vi "TDMS Display File.vi"() -> ()   [LabVIEW 2014]
doc: "Reads Channel groups from a storage."
panel:
  in  "Tab Control":enum32{"Graphs", "Text"}(tab)
  out "ADC Graph & Sensitivity":cluster{dbl, dbl, dbl, dbl, dbl}[](graph)=[{0.6939202535855351, 0.6597435304346917, 0.7798494996227666, 0.7113758520027016, 0.041666666666666664}, {0.7732833719705785, 0.6831987858579877, 0.7047989808668466, 0.7000130127327059, 0.041666666666666664}, {0.7041007332325139, 0.6748832071166728, 0.7563758628274665, 0.7023418195101918, 0.041666666666666664}, {0.7287710343361812, 0.6927783915812504, 0.7367118468836872, 0.7748980582895691, 0.041666666666666664}, {0.6905208333838971, 0.747533064441799, 0.7260319680668351, 0.7577968684325942, 0.041666666666666664}, {0.7790184565798852, 0.7089789165824457, 0.7869391330757264, 0.7335479682280418, 0.041666666666666664}, {0.7547574725819008, 0.6794186579039788, 0.7263648203122135, 0.7405852344135999, 0.041666666666666664}, {0.7856012252236705, 0.7164541312349011, 0.7321340500218805, 0.7793940620799212, 0.041666666666666664}, {0.7863694695366785, 0.7192010621853371, 0.7529441881051713, 0.7942795552898763, 0.041666666666666664}, {0.7143802793590173, 0.7267824228941477, 0.7533863587388494, 0.7549754653750381, 0.041666666666666664}, {0.6889570460159845, 0.6978171767970807, 0.752604474645387, 0.7974266882348474, 0.041666666666666664}, {0.7348739186447792, 0.7511512488908724, 0.7862275846371153, 0.7697490282132154, 0.041666666666666664}, {0.7366489816305779, 0.7076468412533097, 0.7941746731939553, 0.7431999420022006, 0.041666666666666664}, {0.7437110525923172, 0.7293183326362236, 0.7328337328163285, 0.7755590941734851, 0.041666666666666664}, {0.754297094768359, 0.7342720364474336, 0.7253119766780587, 0.707530199890292, 0.041666666666666664}, {0.7718793380822023, 0.7305908805566939, 0.777290626488686, 0.7061421406556109, 0.041666666666666664}, {0.7115328838296461, 0.7639583343927541, 0.7103041909758872, 0.7799545729746497, 0.041666666666666664}, {0.7580782799362614, 0.7922444595666327, 0.793582490808957, 0.7164928001393474, 0.041666666666666664}, {0.7209935129318416, 0.7069085518092215, 0.7276454877529765, 0.7347196698830953, 0.041666666666666664}, {0.7072631490766665, 0.7059021200829305, 0.7059235489574393, 0.7928329938510451, 0.041666666666666664}, {0.7558665739764943, 0.783417340400808, 0.7186483662817867, 0.7048531032784096, 0.041666666666666664}, {0.7259888720514239, 0.7827058907882586, 0.7856346509265696, 0.7319576523845315, 0.041666666666666664}, {0.74059829235442, 0.7286867909911054, 0.740318109215077, 0.7529248645791811, 0.041666666666666664}, {0.7356353131734163, 0.7288697068745372, 0.7176850318597146, 0.7717892323258992, 0.041666666666666664}, {0.7173257455525135, 0.7096572295115393, 0.7672636644207551, 0.7931343209935473, 0.041666666666666664}, {0.7728690641585468, 0.7481594582172137, 0.7986948039298276, 0.7227590658562968, 0.041666666666666664}, {0.7240581644010037, 0.7434758157386584, 0.7939639460929329, 0.7796933777948981, 0.041666666666666664}, {0.0, 0.0, 0.0, 0.0, 0.041666666666666664}, {0.0, 0.0, 0.0, 0.0, 0.041666666666666664}, {0.0, 0.0, 0.0, 0.0, 0.041666666666666664}, {0.0, 0.0, 0.0, 0.0, 0.041666666666666664}, {0.0, 0.0, 0.0, 0.0, 0.041666666666666664}, {0.0, 0.0, 0.0, 0.0, 0.041666666666666664}, {0.7755518153902545, 0.7104068769947832, 0.7404803041697349, 0.7571889248547118, 0.041666666666666664}, {0.7149365159428147, 0.7562761667080153, 0.7655658082814235, 0.7546614486574645, 0.041666666666666664}, {0.7212787265758981, 0.7847814585899867, 0.7008701060788964, 0.744848024239413, 0.041666666666666664}, {0.7539590861913611, 0.7362412923320947, 0.7225911968588279, 0.7072678582111586, 0.041666666666666664}, {0.7457332369970215, 0.7772592809738016, 0.7258779848130176, 0.7997742018754828, 0.041666666666666664}, {0.7462202544308557, 0.7595734610688903, 0.7956340843626722, 0.7482255973738333, 0.041666666666666664}, {0.7892949237206847, 0.7338521115039054, 0.7796435247051742, 0.7289646531269393, 0.041666666666666664}, {0.7894512728814828, 0.7582215635979696, 0.7031641919165742, 0.713359715695722, 0.041666666666666664}, {0.7801688183124195, 0.7810196748023058, 0.78113300185513, 0.7321256124215014, 0.041666666666666664}, {0.7724444570393036, 0.7626952195833875, 0.7612535051718013, 0.7636797337587992, 0.041666666666666664}, {0.726193836599923, 0.7025715443395366, 0.7600099653021122, 0.7575978173214227, 0.041666666666666664}, {0.6928599602194575, 0.7798772159854377, 0.7597272438553717, 0.7812075005180638, 0.041666666666666664}, {0.781487809210651, 0.7612062064634987, 0.7218990796443885, 0.7797000424620804, 0.041666666666666664}, {0.7166320541009918, 0.7834263100440512, 0.7678515500809588, 0.7922811439738483, 0.041666666666666664}, {0.7182030947763013, 0.7910931020099308, 0.7851472394092485, 0.7439923396870723, 0.041666666666666664}, {0.6907666179203221, 0.7377810110090649, 0.7810427433401166, 0.7818706862200796, 0.041666666666666664}, {0.7312453712449207, 0.7490604024135352, 0.7532586729256394, 0.7147550021471913, 0.041666666666666664}, {0.7456867608830217, 0.7451360478820621, 0.7931037481358184, 0.767108452826512, 0.041666666666666664}, {0.6951815348463707, 0.7936814204460578, 0.7633267272309218, 0.7942657913383232, 0.041666666666666664}, {0.7553828225357224, 0.7568992495449439, 0.7345922136156305, 0.771588151980189, 0.041666666666666664}, {0.7429695767133445, 0.765897743360358, 0.7634684516022431, 0.7894448586489562, 0.041666666666666664}, {0.7399032091425222, 0.7288032440908395, 0.7303765797296764, 0.7566677502770919, 0.041666666666666664}, {0.7211293560307285, 0.7179158627748919, 0.7554406467422284, 0.7120925129215225, 0.041666666666666664}, {0.7523970348492739, 0.765370991389381, 0.7434740118117725, 0.766108449040928, 0.041666666666666664}, {0.7121501268469138, 0.7925882050278492, 0.751466109048222, 0.7523113271043922, 0.041666666666666664}, {0.7856519081186785, 0.754151490769755, 0.7261868017394744, 0.7186521662932761, 0.041666666666666664}, {0.7761293635703304, 0.7289798730469097, 0.7218306996500045, 0.7038676590417627, 0.041666666666666664}, {0.7179191679481689, 0.7182690162819555, 0.7444122025372735, 0.7067525552015262, 0.041666666666666664}, {0.7391717580052206, 0.7194903373318009, 0.7069946452929429, 0.7628273895478763, 0.041666666666666664}, {0.7528873020695526, 0.7283262360845427, 0.7325000693073801, 0.7327186254922717, 0.041666666666666664}, {0.7627377902903003, 0.7121581200366729, 0.7774356361278989, 0.7864987984211413, 0.041666666666666664}, {0.7614706971450383, 0.7693062686373836, 0.7596520780174131, 0.791453120693149, 0.041666666666666664}, {0.7758676354288726, 0.7329821109544447, 0.7391832844496626, 0.7040621948075004, 0.041666666666666664}, {0.7485651313430548, 0.7218336773536471, 0.7795020189288245, 0.7853101355604608, 0.041666666666666664}, {0.7977503651267112, 0.7593770002282237, 0.7246274031916076, 0.781837212070119, 0.041666666666666664}, {0.7273354149998054, 0.7406129618939882, 0.7473330540821154, 0.7433034517255335, 0.041666666666666664}, {0.7648587772973705, 0.7253507610953411, 0.7915188498462815, 0.7809612467240841, 0.041666666666666664}, {0.7909263018147277, 0.7309183057278329, 0.7000539453979222, 0.701566380552961, 0.041666666666666664}, {0.7719463781719988, 0.7756144498861192, 0.7748605139353143, 0.711833830053124, 0.041666666666666664}, {0.7522821554311848, 0.7941048840894853, 0.7812308538741344, 0.7367902396056907, 0.041666666666666664}, {0.7866854434339422, 0.7904040217561459, 0.786572030675636, 0.7515730253597176, 0.041666666666666664}, {0.7431088687650106, 0.7826296546335783, 0.742585319011906, 0.767182141229277, 0.041666666666666664}, {0.7628229055220703, 0.7520591249139157, 0.7931985520375183, 0.7451458835282231, 0.041666666666666664}, {0.716552177079085, 0.7927089139381129, 0.7577622400472642, 0.7977649378310769, 0.041666666666666664}, {0.708528438337556, 0.707471228807087, 0.7671195999021296, 0.7596502790257245, 0.041666666666666664}, {0.7255377083440769, 0.7283264739729112, 0.7012629971681663, 0.7881931793708195, 0.041666666666666664}, {0.7166590421880428, 0.7183948555292896, 0.7931008558115896, 0.7010772209591309, 0.041666666666666664}, {0.7600625968935042, 0.7244956222335572, 0.752396089672624, 0.7516733687841425, 0.041666666666666664}, {0.71084210554201, 0.735660980564117, 0.7222812162595661, 0.7370424814051276, 0.041666666666666664}, {0.7281773525093489, 0.7025501267298878, 0.7435778600354459, 0.7594209718616234, 0.041666666666666664}, {0.7507708779236648, 0.7466706425110812, 0.7467961834606034, 0.7532602084876552, 0.041666666666666664}, {0.7331378215250902, 0.7690824168048302, 0.7419505671874272, 0.7847182031732947, 0.08333333333333333}, {0.7663900674619695, 0.732831972277527, 0.7091270673435227, 0.704576265161799, 0.125}, {0.7625782253183676, 0.7744159315624022, 0.7836810871865778, 0.77025187606171, 0.03571428571428571}, {0.7662700014377278, 0.7364215860482902, 0.7977560421751317, 0.7046744970371753, 0.019230769230769232}, {0.7023419054532284, 0.7445916524990491, 0.7783197623813431, 0.7718046969464623, 0.017857142857142856}, {0.7940522278437301, 0.7355956777127955, 0.7056827914859263, 0.7699640310025585, 0.03125}, {0.770151412505229, 0.7787470380637564, 0.7701937621436273, 0.7120881251288848, 0.027777777777777776}, {0.7590860680135483, 0.7193515506620416, 0.7482624622113545, 0.7734007737662043, 0.027777777777777776}, {0.7902528716694006, 0.7920635472066051, 0.7061816422974638, 0.7136584188346482, 0.027777777777777776}, {0.7202475273918132, 0.7120728463926694, 0.7099410165077542, 0.7532619723321432, 0.027777777777777776}, {0.7280834311921148, 0.7222543761195239, 0.7752711117539064, 0.7844367655326663, 0.019230769230769232}, {0.7216642070556465, 0.7808386057862613, 0.7269832478590368, 0.7098337925845678, 0.019230769230769232}, {0.7258473468243719, 0.7867000147035547, 0.7901203071285353, 0.7749291489590999, 0.019230769230769232}, {0.7114154074948261, 0.7237034251052005, 0.7768628688354834, 0.7038342654847397, 0.019230769230769232}, {0.776992432147979, 0.7236427920421763, 0.7156948815630676, 0.7884477458876853, 0.013888888888888888}, {0.7827571632521982, 0.7584136008022355, 0.7273492175968963, 0.7662182461929385, 0.013888888888888888}, {0.7183822940750804, 0.746836694478358, 0.7624403222602808, 0.7375898553279964, 0.013888888888888888}, {0.7466792322952455, 0.7752572572433142, 0.7394298853231326, 0.7539515082977921, 0.013888888888888888}, {0.7413928347892835, 0.739015145244675, 0.719535040118229, 0.7995292148267662, 0.013888888888888888}, {0.744576008173865, 0.7435091818234738, 0.7619895596040774, 0.704510502436212, 0.013888888888888888}, {0.7338843271690502, 0.7301459829714548, 0.7516659017287741, 0.7116540086058052, 0.013888888888888888}, {0.7157306194086261, 0.739270530701973, 0.7384527479670627, 0.7635141296986823, 0.013888888888888888}, {0.7927694855533823, 0.7293486704071075, 0.767631027356994, 0.7624067749388849, 0.013888888888888888}, {0.760568663221189, 0.7870702738129487, 0.7180398074034551, 0.7373794865012128, 0.013888888888888888}, {0.0, 0.0, 0.0, 0.0, 0.013888888888888888}]
  out "Motors & Loopback & Clouds":cluster{dbl, dbl, dbl, dbl, dbl, dbl}[](graph)=[{1.0, 0.0, 1.0, 0.0, 1.0, 1.0}, {0.0, 1.0, 0.0, 0.0, 1.0, 1.0}, {1.0, 0.0, 0.0, 0.0, 1.0, 1.0}, {0.0, 0.0, 1.0, 0.0, 1.0, 1.0}, {0.0, 0.0, 0.0, 0.0, 1.0, 1.0}, {0.0, 0.0, 0.0, 0.0, 1.0, 1.0}, {0.0, 0.0, 1.0, 0.0, 1.0, 1.0}, {0.0, 1.0, 1.0, 0.0, 1.0, 1.0}, {0.0, 0.0, 1.0, 0.0, 1.0, 1.0}, {0.0, 0.0, 0.0, 0.0, 1.0, 1.0}, {1.0, 0.0, 1.0, 0.0, 1.0, 1.0}, {1.0, 0.0, 0.0, 0.0, 1.0, 1.0}, {1.0, 0.0, 0.0, 0.0, 1.0, 1.0}, {0.0, 0.0, 1.0, 0.0, 1.0, 1.0}, {0.0, 0.0, 0.0, 0.0, 1.0, 1.0}, {0.0, 0.0, 0.0, 0.0, 1.0, 1.0}, {0.0, 0.0, 0.0, 0.0, 1.0, 1.0}, {0.0, 0.0, 0.0, 1.0, 1.0, 1.0}, {0.0, 0.0, 0.0, 0.0, 1.0, 1.0}, {0.0, 0.0, 0.0, 0.0, 0.0, 1.0}, {0.0, 0.0, 0.0, 0.0, 0.0, 1.0}, {0.0, 0.0, 0.0, 0.0, 0.0, 1.0}, {0.0, 0.0, 0.0, 0.0, 0.0, 1.0}, {0.0, 0.0, 0.0, 0.0, 0.0, 1.0}, {0.0, 0.0, 0.0, 0.0, 0.0, 1.0}, {0.0, 0.0, 0.0, 0.0, 0.0, 1.0}, {0.0, 0.0, 0.0, 0.0, 0.0, 1.0}, {0.0, 0.0, 0.0, 0.0, 0.0, 1.0}, {0.0, 0.0, 0.0, 0.0, 0.0, 1.0}, {0.0, 0.0, 0.0, 0.0, 0.0, 1.0}, {0.0, 0.0, 0.0, 0.0, 0.0, 1.0}, {0.0, 0.0, 0.0, 0.0, 0.0, 1.0}, {0.0, 0.0, 0.0, 0.0, 0.0, 1.0}, {0.0, 0.0, 0.0, 0.0, 0.0, 1.0}, {0.0, 0.0, 0.0, 0.0, 0.0, 1.0}, {0.0, 0.0, 0.0, 0.0, 0.0, 1.0}, {0.0, 0.0, 0.0, 0.0, 0.0, 1.0}, {0.0, 0.0, 0.0, 0.0, 0.0, 1.0}, {0.0, 0.0, 0.0, 0.0, 0.0, 1.0}, {0.0, 0.0, 0.0, 0.0, 0.0, 1.0}, {0.0, 1.0, 0.0, 1.0, 1.0, 1.0}, {0.0, 0.0, 0.0, 1.0, 1.0, 1.0}, {0.0, 0.0, 0.0, 0.0, 1.0, 1.0}, {0.0, 0.0, 1.0, 0.0, 1.0, 1.0}, {1.0, 0.0, 0.0, 0.0, 1.0, 1.0}, {0.0, 1.0, 0.0, 0.0, 1.0, 1.0}, {1.0, 0.0, 0.0, 0.0, 1.0, 1.0}, {1.0, 0.0, 0.0, 1.0, 1.0, 1.0}, {1.0, 0.0, 1.0, 0.0, 1.0, 1.0}, {0.0, 0.0, 0.0, 0.0, 1.0, 1.0}, {1.0, 0.0, 0.0, 0.0, 1.0, 1.0}, {1.0, 0.0, 0.0, 0.0, 1.0, 1.0}, {0.0, 0.0, 0.0, 0.0, 1.0, 1.0}, {0.0, 0.0, 0.0, 0.0, 1.0, 1.0}, {0.0, 0.0, 0.0, 0.0, 1.0, 1.0}, {0.0, 0.0, 0.0, 0.0, 0.0, 1.0}, {0.0, 0.0, 0.0, 0.0, 0.0, 1.0}, {0.0, 0.0, 0.0, 0.0, 0.0, 1.0}, {0.0, 0.0, 0.0, 0.0, 0.0, 1.0}, {0.0, 0.0, 0.0, 0.0, 0.0, 1.0}, {0.0, 0.0, 0.0, 0.0, 0.0, 1.0}, {0.0, 0.0, 0.0, 0.0, 0.0, 1.0}, {0.0, 0.0, 0.0, 0.0, 0.0, 1.0}, {0.0, 0.0, 0.0, 0.0, 0.0, 1.0}, {0.0, 0.0, 0.0, 0.0, 0.0, 1.0}, {0.0, 0.0, 0.0, 0.0, 0.0, 1.0}, {0.0, 0.0, 0.0, 0.0, 0.0, 1.0}, {0.0, 0.0, 0.0, 0.0, 0.0, 1.0}, {0.0, 0.0, 0.0, 0.0, 0.0, 1.0}, {0.0, 0.0, 0.0, 0.0, 0.0, 1.0}, {0.0, 0.0, 0.0, 0.0, 0.0, 1.0}, {0.0, 0.0, 0.0, 0.0, 0.0, 1.0}, {0.0, 0.0, 0.0, 0.0, 0.0, 1.0}, {0.0, 0.0, 0.0, 0.0, 0.0, 1.0}, {0.0, 0.0, 0.0, 0.0, 0.0, 1.0}, {0.0, 0.0, 0.0, 0.0, 0.0, 1.0}, {0.0, 0.0, 0.0, 0.0, 0.0, 1.0}, {0.0, 0.0, 0.0, 0.0, 0.0, 1.0}, {0.0, 0.0, 0.0, 0.0, 0.0, 1.0}, {0.0, 0.0, 0.0, 0.0, 0.0, 1.0}, {0.0, 0.0, 0.0, 0.0, 0.0, 1.0}, {0.0, 0.0, 0.0, 0.0, 0.0, 1.0}, {0.0, 0.0, 0.0, 0.0, 0.0, 1.0}, {0.0, 0.0, 0.0, 0.0, 0.0, 1.0}, {0.0, 0.0, 0.0, 0.0, 0.0, 1.0}, {0.0, 0.0, 0.0, 0.0, 0.0, 1.0}, {0.0, 0.0, 0.0, 0.0, 0.0, 1.0}, {0.0, 0.0, 0.0, 0.0, 0.0, 1.0}, {0.0, 0.0, 0.0, 0.0, 0.0, 1.0}, {0.0, 0.0, 0.0, 0.0, 0.0, 1.0}, {0.0, 0.0, 0.0, 0.0, 0.0, 1.0}, {0.0, 0.0, 0.0, 0.0, 0.0, 1.0}, {0.0, 0.0, 0.0, 0.0, 0.0, 1.0}, {0.0, 0.0, 0.0, 0.0, 0.0, 1.0}, {0.0, 0.0, 0.0, 0.0, 0.0, 1.0}, {0.0, 0.0, 0.0, 0.0, 0.0, 1.0}, {0.0, 0.0, 0.0, 0.0, 0.0, 1.0}, {0.0, 0.0, 0.0, 0.0, 0.0, 1.0}, {0.0, 0.0, 0.0, 0.0, 0.0, 1.0}, {0.0, 0.0, 0.0, 0.0, 0.0, 1.0}, {0.0, 0.0, 0.0, 0.0, 0.0, 1.0}, {0.0, 0.0, 0.0, 0.0, 0.0, 1.0}, {0.0, 0.0, 0.0, 0.0, 0.0, 1.0}, {0.0, 0.0, 0.0, 0.0, 0.0, 1.0}, {0.0, 0.0, 0.0, 0.0, 0.0, 1.0}, {0.0, 0.0, 0.0, 0.0, 0.0, 1.0}, {0.0, 0.0, 0.0, 0.0, 0.0, 1.0}, {0.0, 0.0, 0.0, 0.0, 0.0, 1.0}, {0.0, 0.0, 0.0, 0.0, 0.0, 1.0}]
  out "TIME        ADC0    ADC1    ADC2   ADC3   SENSITIVITY":string[](array[string])
  out "channel name(s)":string[](array[string])
  out "?":variant[](array[variant])
  out "?":string[](array[string])
  # "Original FP"
  # "File properties"
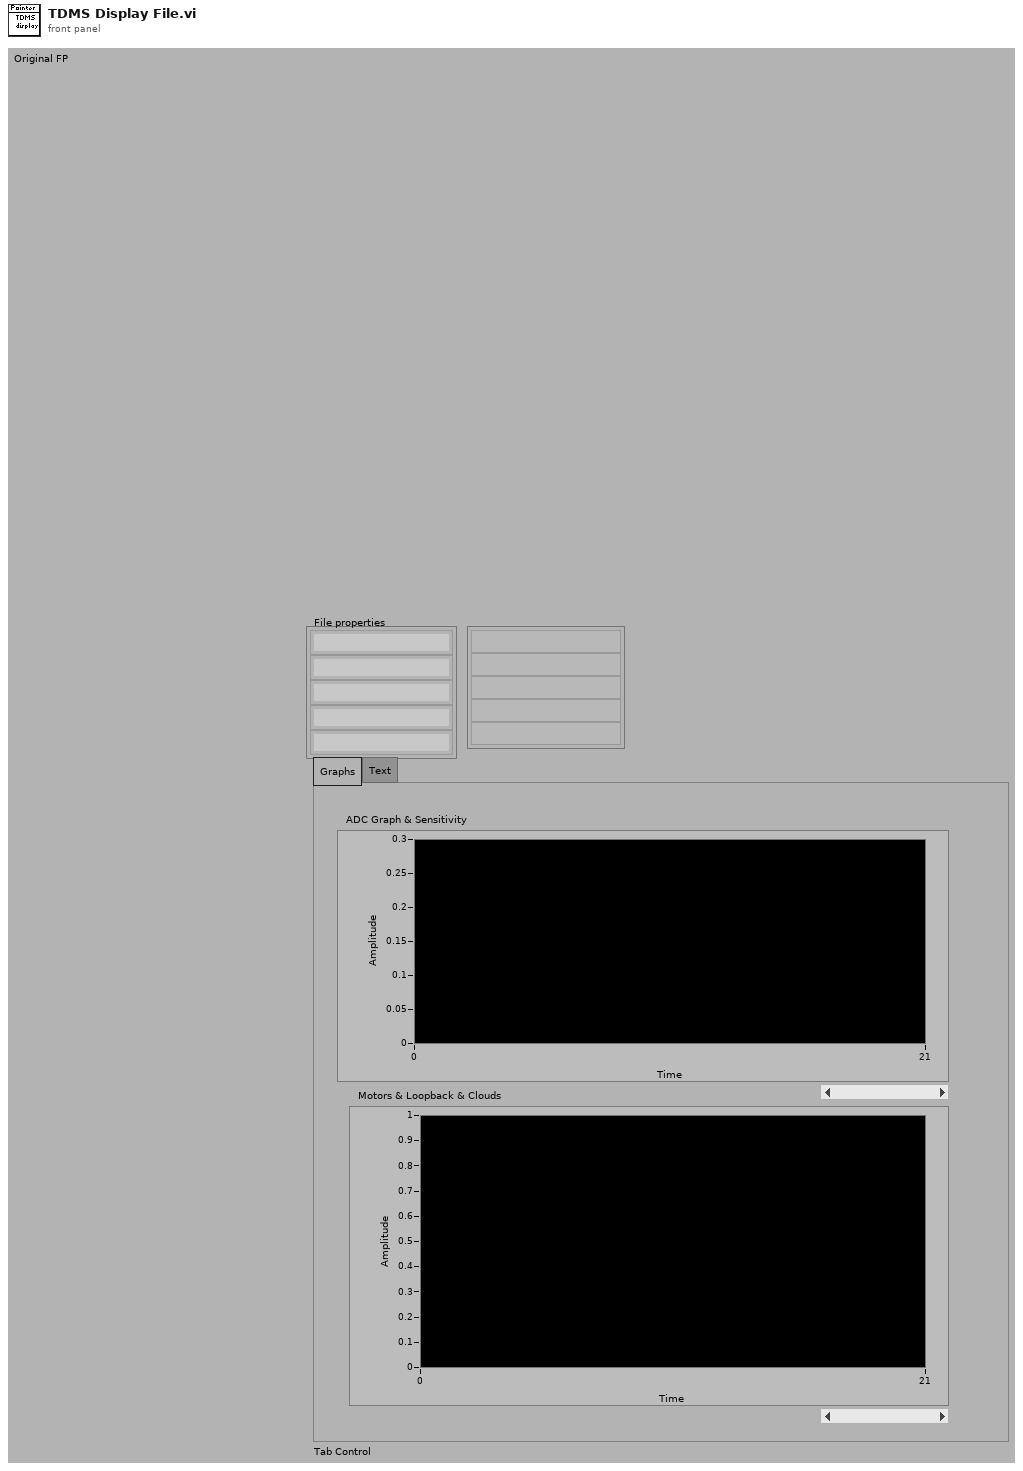
[diagram p1: front panel]
types:
  T1 = enum16{"open", "open or create", "create or replace", "create", "open (read-only)"}
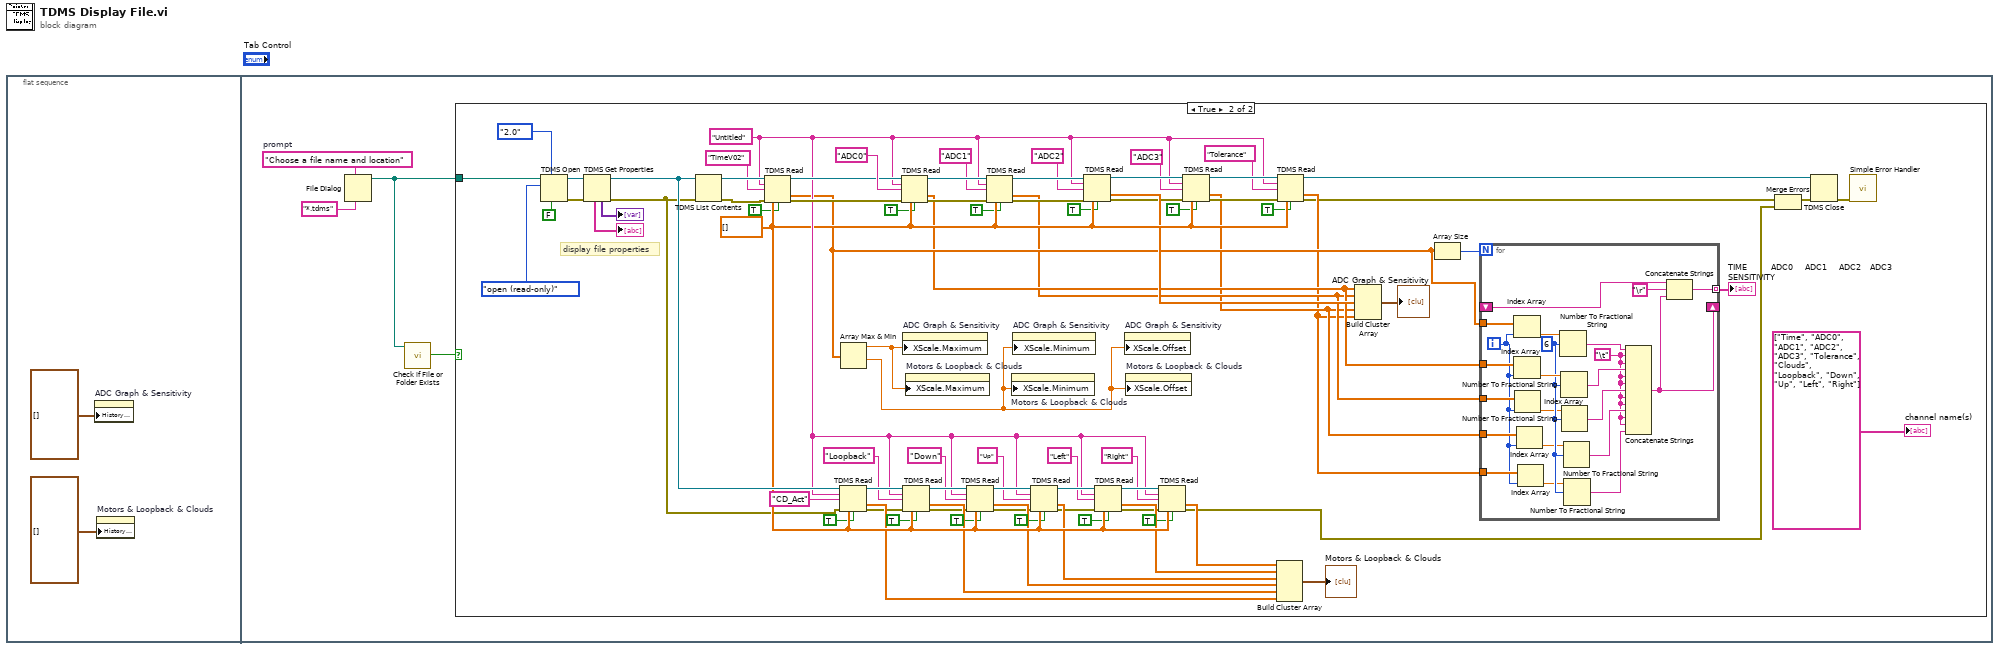
[diagram p0: block diagram]
diagram:
  n1 = flat-sequence {
    frame #0 {
      n2 = property on="ADC Graph & Sensitivity" class="WFChart (strict)"("History Data"=cluster{dbl, dbl, dbl, dbl, dbl}[] []) -> ()  [unwired: 2 in, 2 out]
      n3 = property on="Motors & Loopback & Clouds" class="WFChart (strict)"("History Data"=cluster{dbl, dbl, dbl, dbl, dbl, dbl}[] []) -> ()  [unwired: 2 in, 2 out]
    }
    frame #1 {
      w6 = "Choose a file name and location"  # prompt
      n4 = File Dialog(6:"*.tdms" ("pattern (all files)"), 7:w6) -> (3:w4:path)  [unwired: 1 in, 7 out]
      n5 = call <vilib>:"Check if File or Folder Exists.vi"("path"=w4) -> ("file or folder exists?"=w3:bool)  [unwired: 8 in, 2 out]
      n6 = case shown="True" w3 {
        tunnel: w4 -> [_ w19]
        frame False {
        }
        frame True {
          w48 = dbl[] []
          w54 = "Untitled" ("group name in")
          # "display file properties"
          n7 = TDMS Open(6:FALSE ("disable buffering (T)"), 7:enum16{"1.0", "2.0"}."2.0" ("file format version (2.0)"), 10:T1."open (read-only)" ("operation"), 11:w19) -> (0:w30:errorcluster, 3:w84:refnum<k34>)  [unwired: 3 in]
          n8 = TDMS Get Properties(8:w30, 11:w84) -> (0:w28:errorcluster, 3:w61:refnum<k34>, 4:→"?":variant[], 6:→"?":string[])  [unwired: 6 out]
          n9 = TDMS List Contents(4:w28, 7:w61) -> (0:w73:errorcluster, 3:w81:refnum<k34>)  [unwired: 3 out]
          n10 = TDMS Read(0:w81, 5:w54, 7:"TimeV02" ("channel name(s) in"), 11:w73, 12:w48, 13:TRUE ("return channels in file order? (F)")) -> (4:w67:refnum<k34>, 10:w35:dbl[], 15:w72:errorcluster)  [unwired: 2 in, 3 out]
          n11 = TDMS Read(0:w61, 5:w54, 7:"CD_Act" ("channel name(s) in"), 11:w28, 12:w48, 13:TRUE ("return channels in file order? (F)")) -> (4:w59:refnum<k34>, 10:w42:dbl[], 15:w27:errorcluster)  [unwired: 2 in, 3 out]
          n12 = Array Max & Min(array=w35) -> (max value=w40:dbl, min value=w39:dbl)  [unwired: 2 out]
          n13 = TDMS Read(0:w67, 5:w54, 7:"ADC0" ("channel name(s) in"), 11:w72, 12:w48, 13:TRUE ("return channels in file order? (F)")) -> (4:w78:refnum<k34>, 10:w34:dbl[], 15:w71:errorcluster)  [unwired: 2 in, 3 out]
          n14 = property on="ADC Graph & Sensitivity" class="WFChart (strict)"("XScale.Maximum"=w40) -> ()  [unwired: 2 in, 2 out]
          n15 = TDMS Read(0:w59, 5:w54, 7:"Loopback" ("channel name(s) in"), 11:w27, 12:w48, 13:TRUE ("return channels in file order? (F)")) -> (4:w58:refnum<k34>, 10:w43:dbl[], 15:w26:errorcluster)  [unwired: 2 in, 3 out]
          n16 = property on="Motors & Loopback & Clouds" class="WFChart (strict)"("XScale.Maximum"=w40) -> ()  [unwired: 2 in, 2 out]
          n17 = TDMS Read(0:w58, 5:w54, 7:"Down" ("channel name(s) in"), 11:w26, 12:w48, 13:TRUE ("return channels in file order? (F)")) -> (4:w57:refnum<k34>, 10:w44:dbl[], 15:w25:errorcluster)  [unwired: 2 in, 3 out]
          n18 = TDMS Read(0:w78, 5:w54, 7:"ADC1" ("channel name(s) in"), 11:w71, 12:w48, 13:TRUE ("return channels in file order? (F)")) -> (4:w77:refnum<k34>, 10:w33:dbl[], 15:w70:errorcluster)  [unwired: 2 in, 3 out]
          n19 = property on="Motors & Loopback & Clouds" class="WFChart (strict)"("XScale.Minimum"=w39) -> ()  [unwired: 2 in, 2 out]
          n20 = property on="ADC Graph & Sensitivity" class="WFChart (strict)"("XScale.Minimum"=w39) -> ()  [unwired: 2 in, 2 out]
          n21 = TDMS Read(0:w57, 5:w54, 7:"Up" ("channel name(s) in"), 11:w25, 12:w48, 13:TRUE ("return channels in file order? (F)")) -> (4:w56:refnum<k34>, 10:w45:dbl[], 15:w24:errorcluster)  [unwired: 2 in, 3 out]
          n22 = TDMS Read(0:w77, 5:w54, 7:"ADC2" ("channel name(s) in"), 11:w70, 12:w48, 13:TRUE ("return channels in file order? (F)")) -> (4:w69:refnum<k34>, 10:w38:dbl[], 15:w29:errorcluster)  [unwired: 2 in, 3 out]
          n23 = TDMS Read(0:w56, 5:w54, 7:"Left" ("channel name(s) in"), 11:w24, 12:w48, 13:TRUE ("return channels in file order? (F)")) -> (4:w55:refnum<k34>, 10:w46:dbl[], 15:w23:errorcluster)  [unwired: 2 in, 3 out]
          n24 = property on="ADC Graph & Sensitivity" class="WFChart (strict)"("XScale.Offset"=w39) -> ()  [unwired: 2 in, 2 out]
          n25 = property on="Motors & Loopback & Clouds" class="WFChart (strict)"("XScale.Offset"=w39) -> ()  [unwired: 2 in, 2 out]
          n26 = TDMS Read(0:w55, 5:w54, 7:"Right" ("channel name(s) in"), 11:w23, 12:w48, 13:TRUE ("return channels in file order? (F)")) -> (10:w47:dbl[], 15:w20:errorcluster)  [unwired: 2 in, 4 out]
          n27 = TDMS Read(0:w69, 5:w54, 7:"ADC3" ("channel name(s) in"), 11:w29, 12:w48, 13:TRUE ("return channels in file order? (F)")) -> (4:w65:refnum<k34>, 10:w32:dbl[], 15:w66:errorcluster)  [unwired: 2 in, 3 out]
          n28 = Build Cluster Array(w47, w46, w45, w44, w43, w42) -> (→"Motors & Loopback & Clouds":cluster{dbl, dbl, dbl, dbl, dbl, dbl}[])
          n29 = TDMS Read(0:w65, 5:w54, 7:"Tolerance", 11:w66, 12:w48, 13:TRUE ("return channels in file order? (F)")) -> (4:w63:refnum<k34>, 10:w31:dbl[], 15:w21:errorcluster)  [unwired: 2 in, 3 out]
          n30 = Build Cluster Array(w34, w33, w38, w32, w31) -> (→"ADC Graph & Sensitivity":cluster{dbl, dbl, dbl, dbl, dbl}[])
          n31 = Array Size(array=w35) -> (size(s)=w37:i32)
          n32 = for {
            N: w37 -> [_]
            tunnel: w35 -> [w110]
            tunnel: w34 -> [w109]
            shift-right: [w103] -> _
            shift-left: _ -> [w104]
            tunnel: [w102] -> w36 mode=indexing
            tunnel: w33 -> [w99]
            tunnel: w32 -> [w98]
            tunnel: w31 -> [w97]
            i -> [w89]
            w100 = i16 6 ("width (-)")
            w91 = "\t"
            n33 = Index Array(array=w110, index=w89) -> (element=w108:dbl)
            n34 = Index Array(array=w109, index=w89) -> (element=w107:dbl)
            n35 = Index Array(array=w99, index=w89) -> (element=w96:dbl)
            n36 = Index Array(array=w98, index=w89) -> (element=w95:dbl)
            n37 = Index Array(array=w97, index=w89) -> (element=w94:dbl)
            n38 = Number To Fractional String(number=w108, width (-)=w100) -> (F-format string=w106:string)  [unwired: 2 in]
            n39 = Number To Fractional String(number=w107, width (-)=w100) -> (F-format string=w101:string)  [unwired: 2 in]
            n40 = Number To Fractional String(number=w96, width (-)=w100) -> (F-format string=w93:string)  [unwired: 2 in]
            n41 = Number To Fractional String(number=w95, width (-)=w100) -> (F-format string=w92:string)  [unwired: 2 in]
            n42 = Number To Fractional String(number=w94, width (-)=w100) -> (F-format string=w90:string)  [unwired: 2 in]
            n43 = Concatenate Strings(w106, w91, w91, w101, w91, w91, w93, w91, w91, w92, w91, w91, w90) -> (w103:string)
            n44 = Concatenate Strings(w104, "\r", w103) -> (w102:string)
          }
          "TIME        ADC0    ADC1    ADC2   ADC3   SENSITIVITY" <- w36
          n45 = Merge Errors(w21, w20) -> (w22:errorcluster)
          n46 = TDMS Close(8:w22, 11:w63) -> (0:w88:errorcluster)  [unwired: 1 out]
          n47 = call <vilib>:"Simple Error Handler.vi"("error in (no error)"=w88) -> ()  [unwired: 1 in, 8 out]
          "channel name(s)" <- string[] ["Time", "ADC0", "ADC1", "ADC2", "ADC3", "Tolerance", "Clouds", "Loopback", "Down", "Up", "Left", "Right"] ("channel name(s) in (Untitled)")
        }
      }
    }
  }
